vi "Close.vi"(8 "error in":errorcluster, 11 "Current Limit in":refnum<class "Current Limit.lvclass">) -> (0 "error out":errorcluster, 3 "Current Limit out":refnum<class "Current Limit.lvclass">)   [LabVIEW 2023, in "Current Limit.lvclass"]
uses:
  Current Limit.lvclass
  Current Limit.lvclass/Current Limit.ctl
  Parents/Limit/Limit.lvclass
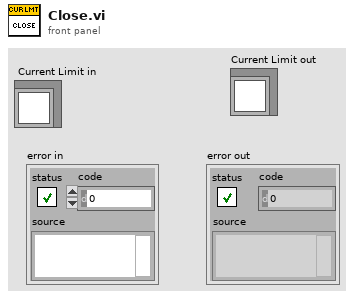
[diagram p1: front panel]
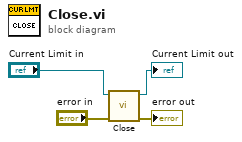
[diagram p0: block diagram]
diagram:
  n1 = call-parent "Close.vi"("error in"="error in", "Limit in"="Current Limit in") -> ("error out"=→"error out":errorcluster, "Limit out"=→"Current Limit out":refnum<class "Current Limit.lvclass">)  [unwired: 8 in]
